vi "PhaseSet.vi"(4 "相位输入":u8[](array[numeric]), 5 "HIFU":bool, 6 "error in (no error)":errorcluster, 7 "chn num":i16=110, 8 "SeqNum":u32, 9 "connection ID in":refnum<k5>) -> (0 "error out":errorcluster, 1 "SeqOUT":u32, 2 "OK?":bool, 3 "connection ID out":refnum<k5>)   [LabVIEW 2016]
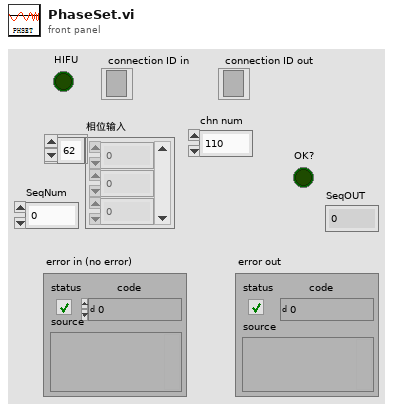
[diagram p1: front panel]
types:
  T1 = enum8{"SET_VOLT", "SET_CHANNEL_VOLT", "SET_PHASE", "START_HEAT", "STOP_HEAT", "CHANNEL_CTRL_SINGLE", "CHANNEL_CTRL_ALL", "READ_VOLT_SET", "READ_VOLT_SET_RSP", "READ_CURRENT_VOLT", "READ_CURRENT_VOLT_RSP", "READ_PHASE", "READ_PHASE_RSP", "READ_HEATTIME_LEFT", "READ_HEATTIME_LEFT_RSP", "EXEC_RSP"}
  T2 = enum8{"SET_VOLT", "SET_CHENNEL_VOLT", "SET_PHASE", "START_HEAT", "STOP_HEAT", "CHANNEL_CTRL_SINGLE", "CHANNEL_CTRL_ALL", "READ_VOLT_SET", "READ_VOLT_SET_RSP", "READ_CURRENT_VOLT", "READ_CURRENT_VOLT_RSP", "READ_PHASE", "READ_PHASE_RSP", "READ_HEATTIME_LEFT", "READ_HEATTIME_LEFT_RSP", "EXEC_RSP"}
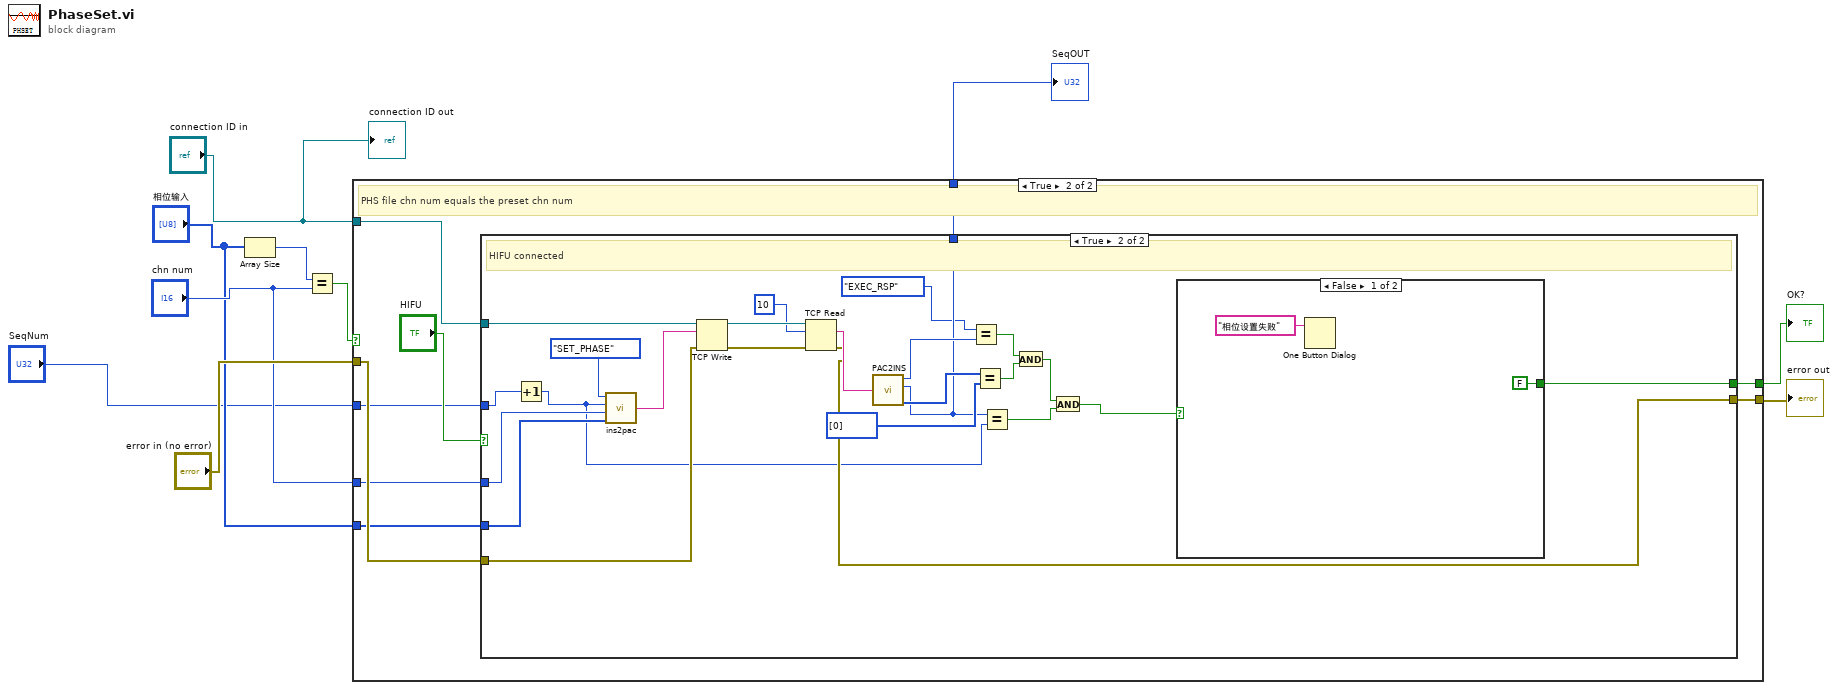
[diagram p0: block diagram]
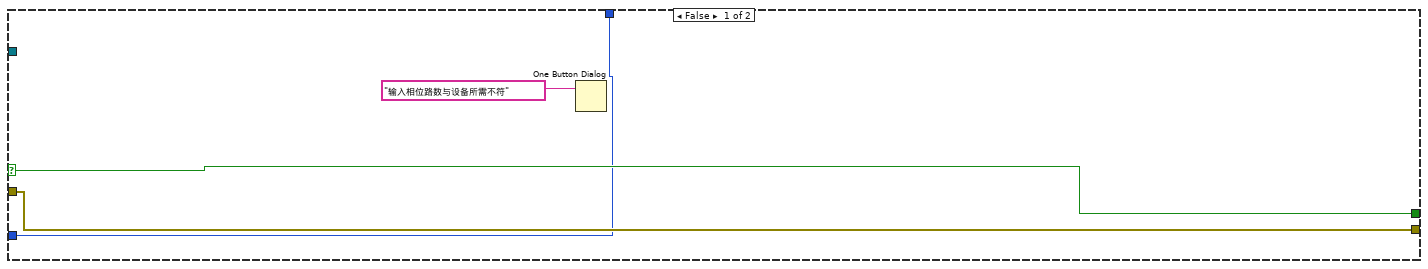
[diagram p2: hidden frame]
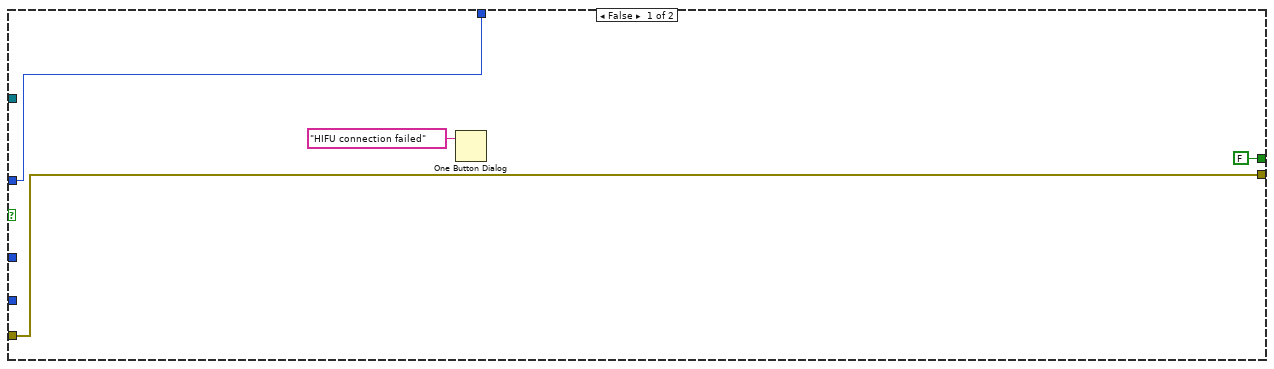
[diagram p3: hidden frame]
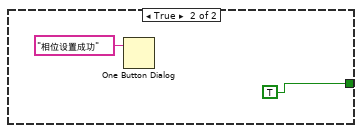
[diagram p4: hidden frame]
diagram:
  n1 = Array Size(array="相位输入") -> (size(s)=w8:i32)
  n2 = Equal?(x=w8, y="chn num") -> (x = y?=w10:bool)
  n3 = case shown="True" w10 {
    selector: w10 -> [w13 _]
    tunnel: "error in (no error)" -> [w12 w22]
    tunnel: [w13 w16] -> w7
    tunnel: [w12 w21] -> w6
    tunnel: "chn num" -> [_ w20]
    tunnel: "相位输入" -> [_ w19]
    tunnel: "SeqNum" -> [w11 w18]
    tunnel: "connection ID in" -> [_ w17]
    tunnel: [w11 w15] -> w1
    frame False {
      n4 = One Button Dialog(message="输入相位路数与设备所需不符") -> ()  [unwired: 1 in, 1 out]
    }
    frame True {
      # "PHS file chn num equals the preset chn num"
      n5 = case shown="True" "HIFU" {
        tunnel: w22 -> [w26 w48]
        tunnel: [w26 w32] -> w21
        tunnel: w20 -> [_ w47]
        tunnel: w19 -> [_ w46]
        tunnel: w18 -> [w24 w31]
        tunnel: w17 -> [_ w50]
        tunnel: [FALSE w33] -> w16
        tunnel: [w24 w29] -> w15
        frame False {
          n6 = One Button Dialog(message="HIFU connection failed") -> ()  [unwired: 1 in, 1 out]
        }
        frame True {
          # "HIFU connected"
          n7 = Increment(x=w31) -> (x+1=w30:u32)
          n8 = call "ins2pac.vi"("BODY"=w46, "chn num"=w47, "SEQUENCE"=w30, "TYPE"=T1."SET_PHASE") -> ("PACKET"=w49:string)
          n9 = TCP Write(connection ID=w50, data in=w49, error in (no error)=w48) -> (connection ID out=w44:refnum<k5>, error out=w45:errorcluster)  [unwired: 1 in, 1 out]
          n10 = TCP Read(connection ID=w44, bytes to read=10, error in (no error)=w45) -> (data out=w42:string, error out=w32:errorcluster)  [unwired: 2 in, 1 out]
          n11 = call "PAC2INS.vi"("PACKET"=w42) -> ("TYPE"=w41:T2, "SEQUENCE"=w29:u32, "BODY"=w39:u8[])  [unwired: 1 out]
          n12 = Equal?(x=T1."EXEC_RSP" ("TYPE"), y=w41) -> (x = y?=w38:bool)
          n13 = Equal?(x=w39, y=i32[] [0]) -> (x = y?=w37:bool)
          n14 = Equal?(x=w29, y=w30) -> (x = y?=w35:bool)
          n15 = And(x=w38, y=w37) -> (x .and. y?=w36:bool)
          n16 = And(x=w36, y=w35) -> (x .and. y?=w34:bool)
          n17 = case shown="False" w34 {
            tunnel: [FALSE TRUE] -> w33
            frame False {
              n18 = One Button Dialog(message="相位设置失败") -> ()  [unwired: 1 in, 1 out]
            }
            frame True {
              n19 = One Button Dialog(message="相位设置成功") -> ()  [unwired: 1 in, 1 out]
            }
          }
        }
      }
    }
  }
  "error out" <- w6
  "OK?" <- w7
  "SeqOUT" <- w1
  "connection ID out" <- "connection ID in"
